vi "MV read status.vi"(8 "error in (no error)":errorcluster, 11 "VISA resource name":refnum<visa-resource-name>="COM1") -> (0 "error out":errorcluster, 2 "status cluster":cluster{"Power (W)":i32, "status indicators":T1} {"status indicators"."Warmed up" scale=0.0..100.0}, 3 "VISA resource name out":refnum<visa-resource-name>)   [LabVIEW 2015, in "Millennia V.lvclass"]
doc: "Reads the current operational status and power of the Millennia V, and checks for any errors."
uses:
  Millennia V.lvclass
  MV status.ctl
  MV warmed up.ctl
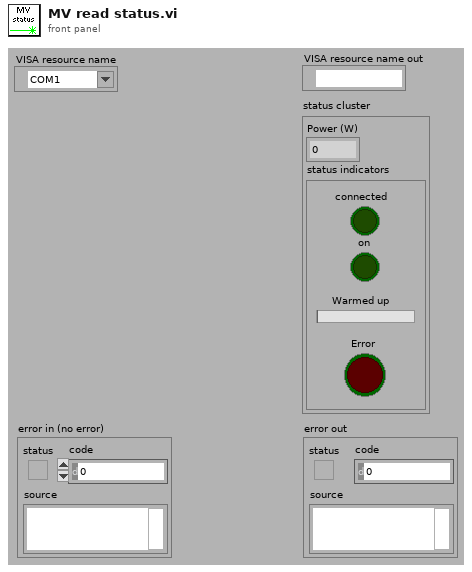
[diagram p1: front panel]
types:
  T1 = typedef "Millennia V.lvclass/MV status.ctl" = cluster{"Millennia V found":bool, "on?":bool, "Error":bool, "Warmed up":T2}
  T2 = typedef "Millennia V.lvclass/MV warmed up.ctl" = dbl
  T3 = enum16{"read only", "write only", "write + read"}
  T4 = cluster{"command error":bool, "execution error":bool, "system error":bool, "laser on":bool, "error":bool, "reserved 1":bool, "reserved 2":bool, "reserved 3":bool}
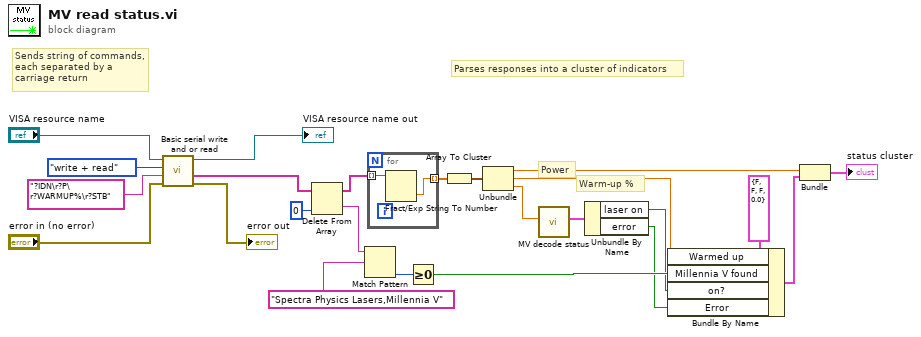
[diagram p0: block diagram]
diagram:
  # "Parses responses into a cluster of indicators"
  # "Sends string of commands, each separated by a carriage return"
  # "Warm-up %"
  # "Power"
  n1 = call "Basic serial write and or read.vi"("error in (no error)"="error in (no error)", "write string"="?IDN\r?P\r?WARMUP%\r?STB", "action"=T3."write + read", "VISA resource name"="VISA resource name") -> ("error out"=→"error out":errorcluster, "read string array"=w12:string[], "VISA resource name out"=→"VISA resource name out":refnum<visa-resource-name>)  [unwired: 4 in, 1 out]
  n2 = Delete From Array(array=w12, index=0) -> (deleted portion=w9:string, array with subset deleted=w11:string[])  [unwired: 1 in]
  n3 = Match Pattern(string=w9, regular expression="Spectra Physics Lasers,Millennia V") -> (offset past match=w13:i32)  [unwired: 1 in, 3 out]
  n4 = for {
    tunnel: w11 -> [w26] mode=indexing
    tunnel: [w25] -> w18 mode=indexing
    n5 = Fract/Exp String To Number(string=w26) -> (number=w25:dbl)  [unwired: 3 in, 1 out]
  }
  n6 = Greater Or Equal To 0?(x=w13) -> (x >= 0?=w5:bool)
  n7 = Array To Cluster(array=w18) -> (cluster=w17:cluster{"[0]":dbl, "[1]":dbl, "[2]":dbl})
  n8 = Unbundle(w17) -> ("[0]"=w8:dbl, "[1]"=w1:dbl, "[2]"=w7:dbl)
  n9 = call "MV decode status.vi"("status byte"=w7) -> ("status cluster"=w16:T4)  [unwired: 10 in]
  n10 = Unbundle By Name(w16) -> ("laser on"=w3:bool, "error"=w4:bool)
  n11 = Bundle By Name(cluster=T1 {"Millennia V found"=FALSE, "on?"=FALSE, "Error"=FALSE, "Warmed up"=0.0} ("status indicators"), "Warmed up"=w1, "Millennia V found"=w5, "on?"=w3, "Error"=w4) -> (w2:T1)
  n12 = Bundle("[0]"=w8, "status indicators"=w2) -> (→"status cluster":cluster{"[0]":dbl, "status indicators":T1})  [unwired: 1 in]
